vi "Teleop.vi"(10 "Match Info":T1={"Autonomous Elapsed Seconds"=0.0, "TeleOp Elapsed Seconds"=0.0, "Disabled Elapsed Seconds"=0.0, "Visited Autonomous"=FALSE, "Visited TeleOp"=FALSE, "Visited Disabled"=FALSE, "Autonomous Settings"={"Autonomous Style"=enum."Independent", "VI Refnum"=refnum}}, 11 "Call Context":T2) -> ()   [LabVIEW 2014]
doc: "This VI is called for each TeleOp packet received from the DS where the robot is not disabled. It is often used to read from the joysticks and update I/O or to update setpoints for timed control loops. It should complete and return within 20 milliseconds or it may miss DS packets."
uses:
  <vilib>/Rock Robotics/WPI/DriverStation/WPI_DriverStationDerivedRobotMode.ctl
  <vilib>/Rock Robotics/WPI/DriverStation/WPI_DriverStationMatch Info.ctl
  <vilib>/Rock Robotics/WPI/RobotDrive/WPI_RobotDriveGetSetRefNum.vi
  <vilib>/Rock Robotics/WPI/Joystick/WPI_JoystickGetSetRefNum.vi
  Robot Global Data.vi
  <vilib>/Rock Robotics/WPI/Ultrasonic/Global 2.vi
panel:
  out "Numeric 1":dbl(slide) scale=0.0..100.0
  out "Boolean 2":bool
  out "Boolean 1":bool
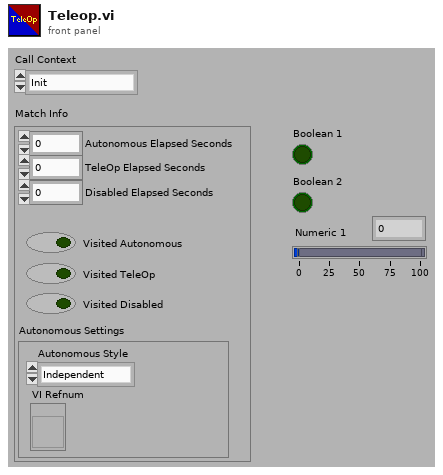
[diagram p1: front panel]
types:
  T1 = typedef "WPI_DriverStationMatch Info.ctl" = cluster{"Autonomous Elapsed Seconds":dbl, "TeleOp Elapsed Seconds":dbl, "Disabled Elapsed Seconds":dbl, "Visited Autonomous":bool, "Visited TeleOp":bool, "Visited Disabled":bool, "Autonomous Settings":cluster{"Autonomous Style":enum16{"Iterative", "Independent"}, "VI Refnum":refnum<vi>}}
  T2 = typedef "WPI_DriverStationDerivedRobotMode.ctl" = enum16{"Init", "Execute", "Stop"}
  T3 = typedef "WPI_JoystickDevRef.ctl" = cluster{"Device":T4}
  T4 = typedef "WPI_JoystickDeviceEnum.ctl" = enum16{"USB 0", "USB 1", "USB 2", "USB 3", "USB 4", "USB 5"}
  T5 = typedef "WPI_EncoderDevRef.ctl" = cluster{"DevStatus":errorcluster, "EncoderIndex":T6, "CounterIndex":T7, "DistancePerCount":dbl, "Decoding Type":T8}
  T6 = typedef "FPGA_EncoderIdx.ctl" = enum8{"Enc 0", "Enc 1", "Enc 2", "Enc 3", "Invalid"}
  T7 = typedef "FPGA_CounterCtrSystemIndex.ctl" = enum8{"Ctr 0", "Ctr 1", "Ctr 2", "Ctr 3", "Ctr 4", "Ctr 5", "Ctr 6", "Ctr 7", "Invalid"}
  T8 = typedef "WPI_EncoderType.ctl" = enum16{"1x", "2x", "4x"}
  T9 = cluster{"Button 1":bool, "Button 2":bool, "Button 3":bool, "Button 4":bool, "Button 5":bool, "Button 6":bool, "Button 7":bool, "Button 8":bool, "Button 9":bool, "Button 10":bool, "Button 11":bool, "Button 12":bool}
  T10 = cluster{"axis 1 (x)":dbl, "axis 2 (y)":dbl, "axis 3 (throttle)":dbl, "axis 4":dbl, "axis 5":dbl, "axis 6":dbl}
  T11 = typedef "WPI_DigitalInputDevRef.ctl" = cluster{"DevStatus":errorcluster, "DIO Channel":T12, "Digital Module":T13}
  T12 = typedef "FPGA_DIOChannel.ctl" = enum8{"DIO 1", "DIO 2", "DIO 3", "DIO 4", "DIO 5", "DIO 6", "DIO 7", "DIO 8", "DIO 9", "DIO 10", "DIO 11", "DIO 12", "DIO 13", "DIO 14", "Invalid"}
  T13 = typedef "FPGA_TypedefDigitalModule.ctl" = enum16{"Digital Module 1", "Digital Module 2"}
  T14 = typedef "WPI_MotorControlDeviceRef.ctl" = cluster{"DeviceStatus":errorcluster, "Type":enum16{"PWM", "CAN"}, "PWM":cluster{"Digital Module":T13, "PWM Channel":T15, "DeadBand":T16}, "CAN":cluster{"Device Number":u8, "Control Mode":T17, "Semaphore":T18, "Max Vout":dbl}, "Invert":bool, "TransformRef":T19, "InvTransformRef":T19}
  T15 = typedef "FPGA_DIOPWMChannel.ctl" = enum8{"PWM 1", "PWM 2", "PWM 3", "PWM 4", "PWM 5", "PWM 6", "PWM 7", "PWM 8", "PWM 9", "PWM 10", "Invalid"}
  T16 = typedef "WPI_PWMDeadband.ctl" = cluster{"Name":string, "maxPositivePwm":i32, "minPositivePwm":i32, "centerPwm":i32, "maxNegativePwm":i32, "minNegativePwm":i32, "angularRange":u16}
  T17 = typedef "WPI_CANJaguar_ControlMode.ctl" = enum8{"Percent VBus", "Current", "Speed", "Position", "Voltage"}
  T18 = typedef "Semaphore RefNum" = refnum<k1>
  T19 = typedef "WPI_PWMTransform_ConPane.ctl" = refnum<vi>
  T20 = typedef "WPI_RobotDriveDevRef.ctl" = cluster{"DevStatus":errorcluster, "Motors[]":T14[], "Square Inputs":bool, "Max Output":dbl}
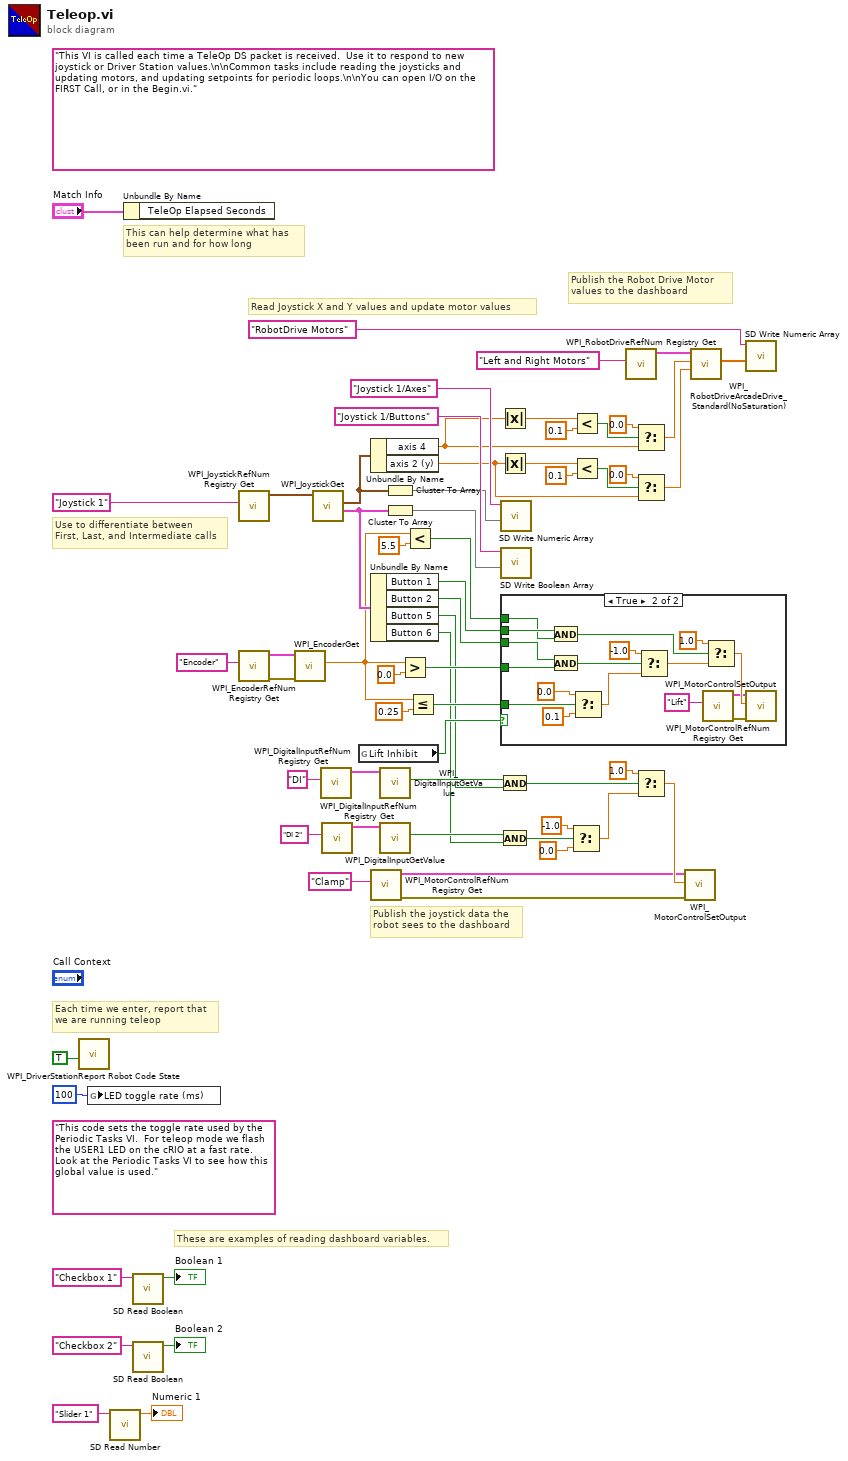
[diagram p0: block diagram]
diagram:
  (unwired) "This code sets the toggle rate used by the Periodic Tasks VI.  For teleop mode we flash the USER1 LED on the cRIO at a fast rate.  Look at the Periodic Tasks VI to see how this global value is used."
  (unwired) "This VI is called each time a TeleOp DS packet is received.  Use it to respond to new joystick or Driver Station values.\n\nCommon tasks include reading the joysticks and updating motors, and updating setpoints for periodic loops.\n\nYou can open I/O on the FIRST Call, or in the Begin.vi."
  # "These are examples of reading dashboard variables."
  # "Publish the Robot Drive Motor\nvalues to the dashboard"
  # "Publish the joystick data the\nrobot sees to the dashboard"
  # "Each time we enter, report that\nwe are running teleop"
  # "Use to differentiate between\nFirst, Last, and Intermediate calls"
  # "This can help determine what has\nbeen run and for how long"
  # "Read Joystick X and Y values and update motor values"
  n1 = call <vilib>:"WPI_DriverStationReport Robot Code State.vi"("TeleOp"=TRUE ("Autonomous")) -> ()  [unwired: 10 in, 1 out]
  n2 = global write "Robot Global Data.vi" "LED toggle rate (ms)"(u32 100 ("LED ms toggle rate")) -> ()
  n3 = call <vilib>:"SD Read Number.vi"("Name"="Slider 1" ("refnum name")) -> ("Numeric"=→"Numeric 1":dbl)  [unwired: 8 in, 2 out]
  n4 = Unbundle By Name("Match Info") -> ()  [unwired: 1 out]
  n5 = call <vilib>:"SD Read Boolean.vi"("Name"="Checkbox 1" ("refnum name")) -> ("Boolean"=→"Boolean 1":bool)  [unwired: 8 in, 2 out]
  n6 = call <vilib>:"SD Read Boolean.vi"("Name"="Checkbox 2" ("refnum name")) -> ("Boolean"=→"Boolean 2":bool)  [unwired: 8 in, 2 out]
  n7 = call <vilib>:"WPI_JoystickRefNum Registry Get.vi"("refnum name"="Joystick 1") -> ("JoystickDevRef"=w60:T3)  [unwired: 1 in, 9 out]
  n8 = call <vilib>:"WPI_EncoderRefNum Registry Get.vi"("refnum name"="Encoder") -> ("error out"=w22:errorcluster, "EncoderDevRef"=w23:T5)  [unwired: 9 in]
  n9 = call <vilib>:"WPI_EncoderGet.vi"("error in (no error)"=w22, "EncoderDevRef"=w23) -> ("Distance"=w13:dbl)  [unwired: 4 in, 5 out]
  n10 = call <vilib>:"WPI_JoystickGet.vi"("JoystickDevRef"=w60) -> ("Buttons"=w32:T9, "Axes"=w55:T10)  [unwired: 1 in, 4 out]
  n11 = call <vilib>:"WPI_DigitalInputRefNum Registry Get.vi"("refnum name"="DI") -> ("DigitalInputDevRef"=w10:T11)  [unwired: 9 in, 1 out]
  n12 = call <vilib>:"WPI_DigitalInputRefNum Registry Get.vi"("refnum name"="DI 2") -> ("DigitalInputDevRef"=w8:T11)  [unwired: 9 in, 1 out]
  n13 = global read "Global 2.vi" "Lift Inhibit"() -> (w11:bool)
  n14 = Unbundle By Name(w55) -> ("axis 4"=w35:dbl, "axis 2 (y)"=w40:dbl)
  n15 = Unbundle By Name(w32) -> ("Button 1"=w20:bool, "Button 2"=w19:bool, "Button 5"=w5:bool, "Button 6"=w2:bool)
  n16 = call <vilib>:"WPI_MotorControlRefNum Registry Get.vi"("refnum name"="Clamp") -> ("error out"=w26:errorcluster, "MotorControlDevRef"=w25:T14)  [unwired: 9 in]
  n17 = call <vilib>:"WPI_DigitalInputGetValue.vi"("DigitalInputDevRef"=w10) -> ("Value"=w6:bool)  [unwired: 8 in, 2 out]
  n18 = call <vilib>:"WPI_DigitalInputGetValue.vi"("DigitalInputDevRef"=w8) -> ("Value"=w3:bool)  [unwired: 8 in, 2 out]
  n19 = Cluster To Array(cluster=w55) -> (array=w54:dbl[])
  n20 = Cluster To Array(cluster=w32) -> (array=w57:bool[])
  n21 = Greater?(x=w13, y=0.0) -> (0:w17:bool)
  n22 = Less?(x=w13, y=5.5) -> (x < y?=w15:bool)
  n23 = Less Or Equal?(x=w13, y=0.25) -> (x <= y?=w14:bool)
  n24 = Absolute Value(x=w35) -> (abs(x)=w39:dbl)
  n25 = Absolute Value(x=w40) -> (abs(x)=w44:dbl)
  n26 = And(x=w6, y=w5) -> (x .and. y?=w4:bool)
  n27 = And(x=w3, y=w2) -> (x .and. y?=w1:bool)
  n28 = call <vilib>:"SD Write Numeric Array.vi"("Numeric Array"=w54, "Name"="Joystick 1/Axes") -> ()  [unwired: 8 in, 2 out]
  n29 = call <vilib>:"SD Write Boolean Array.vi"("Boolean Array"=w57, "Name"="Joystick 1/Buttons") -> ()  [unwired: 8 in, 2 out]
  n30 = case shown="True" w11 {
    tunnel: w20 -> [_ w74]
    tunnel: w19 -> [_ w73]
    tunnel: w17 -> [_ w72]
    tunnel: w15 -> [_ w69]
    tunnel: w14 -> [_ w67]
    frame False {
    }
    frame True {
      n31 = And(x=w74, y=w69) -> (x .and. y?=w70:bool)
      n32 = And(x=w73, y=w72) -> (x .and. y?=w71:bool)
      n33 = Select(t=0.0, s=w67, f=0.1) -> (s? t:f=w68:dbl)
      n34 = Select(t=-1.0, s=w71, f=w68) -> (s? t:f=w80:dbl)
      n35 = call <vilib>:"WPI_MotorControlRefNum Registry Get.vi"("refnum name"="Lift") -> ("error out"=w77:errorcluster, "MotorControlDevRef"=w76:T14)  [unwired: 9 in]
      n36 = Select(t=1.0, s=w70, f=w80) -> (s? t:f=w78:dbl)
      n37 = call <vilib>:"WPI_MotorControlSetOutput.vi"("error in (no error)"=w77, "Output"=w78, "MotorControlDevRef"=w76) -> ()  [unwired: 6 in, 3 out]
    }
  }
  n38 = Select(t=-1.0, s=w1, f=0.0) -> (s? t:f=w30:dbl)
  n39 = Less?(x=w39, y=0.1) -> (x < y?=w37:bool)
  n40 = Less?(x=w44, y=0.1) -> (x < y?=w42:bool)
  n41 = call <vilib>:"WPI_RobotDriveRefNum Registry Get.vi"("refnum name"="Left and Right Motors") -> ("RobotDriveDevRef"=w62:T20)  [unwired: 1 in, 9 out]
  n42 = Select(t=0.0, s=w37, f=w35) -> (s? t:f=w34:dbl)
  n43 = Select(t=0.0, s=w42, f=w40) -> (s? t:f=w33:dbl)
  n44 = Select(t=1.0, s=w4, f=w30) -> (s? t:f=w27:dbl)
  n45 = call <vilib>:"WPI_MotorControlSetOutput.vi"("error in (no error)"=w26, "Output"=w27, "MotorControlDevRef"=w25) -> ()  [unwired: 6 in, 3 out]
  n46 = call <vilib>:"WPI_RobotDriveArcadeDrive_Standard(NoSaturation).vi"("Y axis value"=w33, "X axis value"=w34, "RobotDriveDevRef"=w62) -> ("Motor Values"=w51:dbl[])  [unwired: 1 in, 7 out]
  n47 = call <vilib>:"SD Write Numeric Array.vi"("Numeric Array"=w51, "Name"="RobotDrive Motors") -> ()  [unwired: 8 in, 2 out]
